vi "get_current_vars.vi"(8 "error in (no error)":errorcluster, 11 "ExperimentVariables in":refnum<class "ExperimentVariables.lvclass">) -> (0 "error out":errorcluster, 1 "current variable indicies":i32[](array[numeric]), 2 "variables and parameter names":string[](array[string]), 3 "ExperimentVariables out":refnum<class "ExperimentVariables.lvclass">, 4 "current variable and parameter values":dbl[](array[numeric]), 5 "variable names":string[](array[string]))   [LabVIEW 2012, in "ExperimentVariables.lvclass"]
uses:
  ExperimentVariables.lvclass
  ExperimentVariables.lvclass/ExperimentVariables.ctl
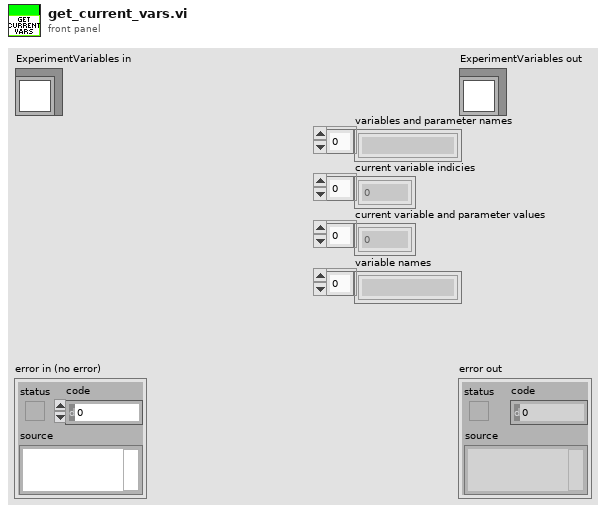
[diagram p1: front panel]
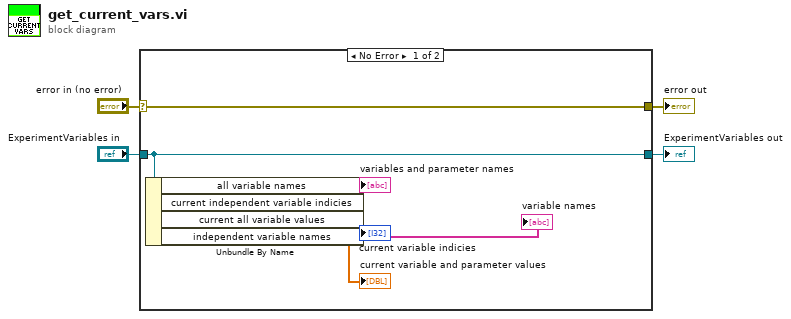
[diagram p0: block diagram]
diagram:
  n1 = case shown="No Error" "error in (no error)" {
    selector: "error in (no error)" -> [w10 w12]
    tunnel: [w10 w12] -> w3
    tunnel: [w9 w11] -> w1
    tunnel: "ExperimentVariables in" -> [w9 w11]
    frame No Error {
      n2 = Unbundle By Name(w9) -> ("all variable names"=→"variables and parameter names":string[], "current independent variable indicies"=→"current variable indicies":i32[], "current all variable values"=→"current variable and parameter values":dbl[], "independent variable names"=→"variable names":string[])
    }
    frame Error {
    }
  }
  "error out" <- w3
  "ExperimentVariables out" <- w1
